vi "SaveTempCalibrLog.vi"() -> (2 "selected path":path, 3 "Boolean":bool)   [LabVIEW 2020]
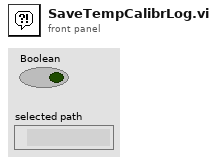
[diagram p1: front panel]
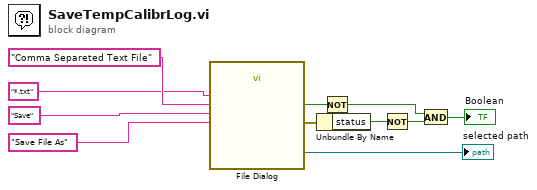
[diagram p0: block diagram]
diagram:
  n1 = call "File Dialog"("prompt"="Save File As", "button label"="Save", "pattern (all files)"="*.txt", "pattern label"="Comma Separeted Text File") -> ("selected path"=→"selected path":path, "cancelled"=w7:bool, "error out"=w5:errorcluster)  [unwired: 8 in, 1 out]
  n2 = Unbundle By Name(w5) -> ("status"=w6:bool)
  n3 = Not(x=w7) -> (.not. x?=w9:bool)
  n4 = Not(x=w6) -> (.not. x?=w8:bool)
  n5 = And(x=w9, y=w8) -> (x .and. y?=→"Boolean":bool)
